vi "HOST Serial thruster update.vi"(8 "error in (no error)":errorcluster, 11 "Data out":T1={"VI References"=[], "Addresses"=[], "Pilot"=FALSE, "DO Data"=[], "Access Restricted?"=FALSE, "Pilot Control References"=[], "CoPilot Control References"=[], "cRIO Config"=[], "datalog Q"=refnum, "PS_P"={"AI"=[], "DI"=[], "DO"=[], "Serial"=[], "CPU"={"Total Load"=[], "Interrupt Load"=[], "Total Physical"=0.0, "Free Physical"=0.0, "Primary Disk Capacity"=0.0, "Primary Disk Free"=0.0}, "Stop"=FALSE, "DO Channel"=[]}, "PS_S"={"AI"=[], "DI"=[], "DO"=[], "Serial"=[], "CPU"={"Total Load"=[], "Interrupt Load"=[], "Total Physical"=0.0, "Free Physical"=0.0, "Primary Disk Capacity"=0.0, "Primary Disk Free"=0.0}, "Stop"=FALSE, "DO Channel"=[]}, "IDE_P"={"AI"=[], "DI"=[], "DO"=[], "Serial"=[], "CPU"={"Total Load"=[], "Interrupt Load"=[], "Total Physical"=0.0, "Free Physical"=0.0, "Primary Disk Capacity"=0.0, "Primary Disk Free"=0.0}, "Stop"=FALSE, "DO Channel"=[]}, "IDE_S"={"AI"=[], "DI"=[], "DO"=[], "Serial"=[], "CPU"={"Total Load"=[], "Interrupt Load"=[], "Total Physical"=0.0, "Free Physical"=0.0, "Primary Disk Capacity"=0.0, "Primary Disk Free"=0.0}, "Stop"=FALSE, "DO Channel"=[]}, "PDE_P"={"AI"=[], "DI"=[], "DO"=[], "Serial"=[], "CPU"={"Total Load"=[], "Interrupt Load"=[], "Total Physical"=0.0, "Free Physical"=0.0, "Primary Disk Capacity"=0.0, "Primary Disk Free"=0.0}, "Stop"=FALSE, "DO Channel"=[]}, "PDE_S"={"AI"=[], "DI"=[], "DO"=[], "Serial"=[], "CPU"={"Total Load"=[], "Interrupt Load"=[], "Total Physical"=0.0, "Free Physical"=0.0, "Primary Disk Capacity"=0.0, "Primary Disk Free"=0.0}, "Stop"=FALSE, "DO Channel"=[]}, "GUI References"={"Control Names"=[], "Control References"=[]}, "GUI Data"=[], "TCP - Serial"=[], "TCP-Serial Q"=refnum, "TCP Serial Ref"=[], "Data Sets"=[], "Last Data"=[], "Alarm Data"=[], "DI Data"=[], "Ack Data"=[], "Buzzer Data"=[], "Pilot DO"=[], "Co-Pilot DO"=[], "System Down?"=FALSE, "Log Data"=[], "Update Array"=[], "MCC Data Log"=[], "MCC Data Not"=refnum, "Thruster control"=[refnum, refnum, refnum, refnum, refnum, refnum, refnum, refnum, refnum], "waga notifier out"=refnum, "Wago  log"=[], "Thruster Cont"=[0.0, 0.0, 0.0, 0.0, 0.0, 0.0, 0.0, 0.0, 0.0], "Cam Cont"=[FALSE, FALSE, FALSE, FALSE, FALSE, TRUE], "PDE_P TH Cont"={"COM 10"=0.0, "COM 11"=0.0, "COM 12"=0.0, "COM 13"=0.0}, "PDE_S TH Cont"={"COM 10"=0.0, "COM 11"=0.0, "COM 12"=0.0, "COM 13"=0.0}} {"cRIO Config"."AI"."Interface Data"."Timing"."sample mode" items=["Finite Samples"=10178, "Continuous Samples"=10123, "Hardware Timed Single Point"=12522]; "cRIO Config"."Async"."Interface Data"."Data"."Minor Frame Count" min=5 max=8 step=1}) -> (0 "error out":errorcluster, 3 "Data out 2":T1={"VI References"=[], "Addresses"=[], "Pilot"=FALSE, "DO Data"=[], "Access Restricted?"=FALSE, "Pilot Control References"=[], "CoPilot Control References"=[], "cRIO Config"=[], "datalog Q"=refnum, "PS_P"={"AI"=[], "DI"=[], "DO"=[], "Serial"=[], "CPU"={"Total Load"=[], "Interrupt Load"=[], "Total Physical"=0.0, "Free Physical"=0.0, "Primary Disk Capacity"=0.0, "Primary Disk Free"=0.0}, "Stop"=FALSE, "DO Channel"=[]}, "PS_S"={"AI"=[], "DI"=[], "DO"=[], "Serial"=[], "CPU"={"Total Load"=[], "Interrupt Load"=[], "Total Physical"=0.0, "Free Physical"=0.0, "Primary Disk Capacity"=0.0, "Primary Disk Free"=0.0}, "Stop"=FALSE, "DO Channel"=[]}, "IDE_P"={"AI"=[], "DI"=[], "DO"=[], "Serial"=[], "CPU"={"Total Load"=[], "Interrupt Load"=[], "Total Physical"=0.0, "Free Physical"=0.0, "Primary Disk Capacity"=0.0, "Primary Disk Free"=0.0}, "Stop"=FALSE, "DO Channel"=[]}, "IDE_S"={"AI"=[], "DI"=[], "DO"=[], "Serial"=[], "CPU"={"Total Load"=[], "Interrupt Load"=[], "Total Physical"=0.0, "Free Physical"=0.0, "Primary Disk Capacity"=0.0, "Primary Disk Free"=0.0}, "Stop"=FALSE, "DO Channel"=[]}, "PDE_P"={"AI"=[], "DI"=[], "DO"=[], "Serial"=[], "CPU"={"Total Load"=[], "Interrupt Load"=[], "Total Physical"=0.0, "Free Physical"=0.0, "Primary Disk Capacity"=0.0, "Primary Disk Free"=0.0}, "Stop"=FALSE, "DO Channel"=[]}, "PDE_S"={"AI"=[], "DI"=[], "DO"=[], "Serial"=[], "CPU"={"Total Load"=[], "Interrupt Load"=[], "Total Physical"=0.0, "Free Physical"=0.0, "Primary Disk Capacity"=0.0, "Primary Disk Free"=0.0}, "Stop"=FALSE, "DO Channel"=[]}, "GUI References"={"Control Names"=[], "Control References"=[]}, "GUI Data"=[], "TCP - Serial"=[], "TCP-Serial Q"=refnum, "TCP Serial Ref"=[], "Data Sets"=[], "Last Data"=[], "Alarm Data"=[], "DI Data"=[], "Ack Data"=[], "Buzzer Data"=[], "Pilot DO"=[], "Co-Pilot DO"=[], "System Down?"=FALSE, "Log Data"=[], "Update Array"=[], "MCC Data Log"=[], "MCC Data Not"=refnum, "Thruster control"=[refnum, refnum, refnum, refnum, refnum, refnum, refnum, refnum, refnum], "waga notifier out"=refnum, "Wago  log"=[], "Thruster Cont"=[0.0, 0.0, 0.0, 0.0, 0.0, 0.0, 0.0, 0.0, 0.0], "Cam Cont"=[FALSE, FALSE, FALSE, FALSE, FALSE, TRUE], "PDE_P TH Cont"={"COM 10"=0.0, "COM 11"=0.0, "COM 12"=0.0, "COM 13"=0.0}, "PDE_S TH Cont"={"COM 10"=0.0, "COM 11"=0.0, "COM 12"=0.0, "COM 13"=0.0}} {"cRIO Config"."AI"."Interface Data"."Timing"."sample mode" items=["Finite Samples"=10178, "Continuous Samples"=10123, "Hardware Timed Single Point"=12522]; "cRIO Config"."Async"."Interface Data"."Data"."Minor Frame Count" min=5 max=8 step=1})   [LabVIEW 2021]
doc: "Thruster control data trnsmission to teh slave will be updated with this Vi. The data will be read from the serial and updated with corresponding to Slave and System Down Status."
uses:
  Controls/Host - GUI Data Cluster.ctl
  Analog Output/Controls/AO JSON Data Cluster.ctl
  Analog Output/Controls/AO Interface Data Cluster.ctl
  Analog Output/Controls/AO Channel Configuration Cluster.ctl
  Analog Output/Controls/AO Timing Cluster.ctl
  Digital Output/Controls/DIO Configuration cluster.ctl
  Digital Output/Controls/DIO Interface Data.ctl
  Digital Output/SubVIs/Digital Dynamic Cluster.ctl
  Async JSON Cluster.ctl
  Async Interface Data Cluster.ctl
  Async Serial/Controls/Async Serial Configuration Cluster.ctl
  Async Serial/Controls/Async Frame Info Cluster.ctl
  Async Serial/Controls/Async Message Info Cluster.ctl
  Controls/Host Data Cluster.ctl
  Main Engine/Controls/Main Engine CPU Info.ctl
panel:
  out "PDE_S.Serial 2":string[][](array[string])
  out "Array":i32[](array[numeric])
  out "PDE_S.Serial":string[][](array[string])=[["com21", "4000.000000", "TRUE", "", "", "", "", "", "", "", "", ""], ["com12", "96.000000", "156.989250", "0.125000", "37.678600", "28.353846", "-138.261345", "19.484347", "0.000000", "0.000000", "0.000000", "0.000000"], ["com13", "96.000000", "157.038750", "0.750000", "37.678025", "28.353846", "21.753627", "19.979010", "0.000000", "0.000000", "0.000000", "0.000000"], ["com10", "96.000000", "157.088250", "0.250000", "37.677450", "31.169231", "22.048668", "20.077840", "0.000000", "0.000000", "0.000000", "0.000000"], ["com11", "96.000000", "157.830750", "0.250000", "37.679175", "30.856410", "20.670168", "20.176638", "0.000000", "0.000000", "0.000000", "0.000000"]]
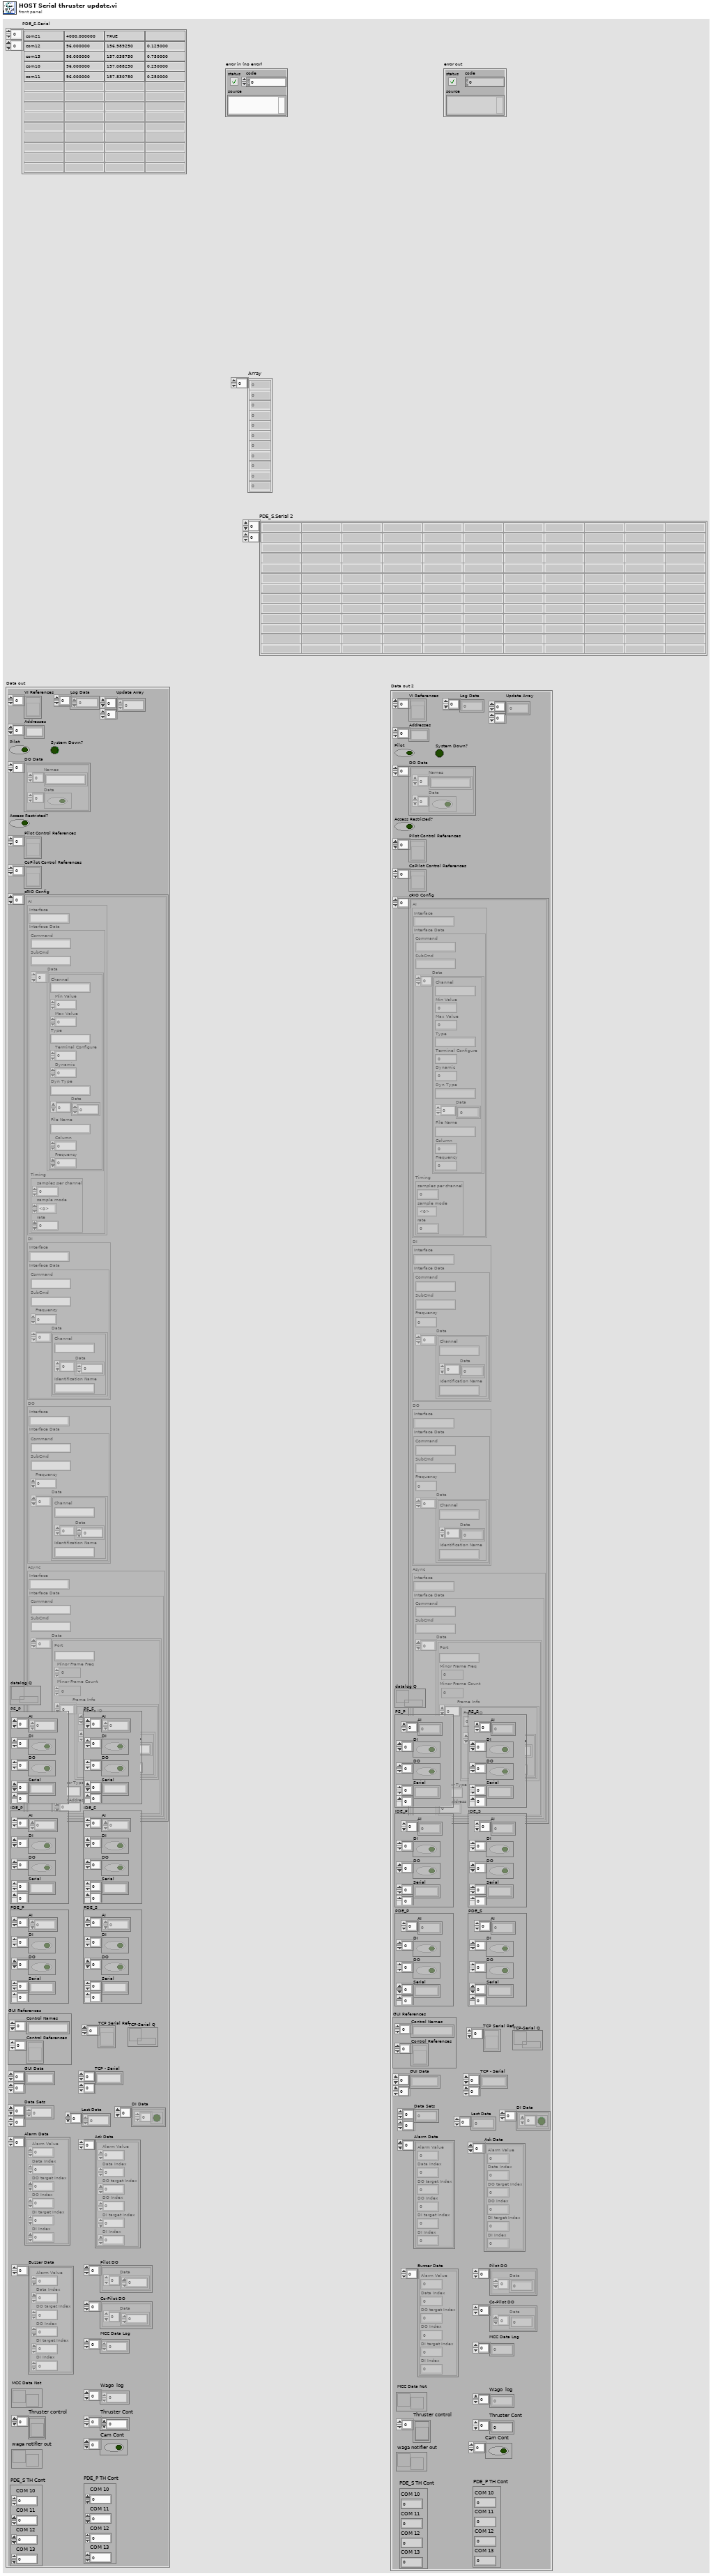
[diagram p1: front panel]
types:
  T1 = typedef "Host - GUI Data Cluster.ctl" = cluster{"VI References":refnum<vi>[], "Addresses":string[], "Pilot":bool, "DO Data":cluster{"Names":string[], "Data":bool[]}[], "Access Restricted?":bool, "Pilot Control References":refnum<vi>[], "CoPilot Control References":refnum<vi>[], "cRIO Config":cluster{"AI":T2, "DI":T6, "DO":T6, "Async":T9}[], "datalog Q":refnum<queue>, "PS_P":T14, "PS_S":T14, "IDE_P":T14, "IDE_S":T14, "PDE_P":T14, "PDE_S":T14, "GUI References":cluster{"Control Names":string[], "Control References":refnum<vi>[]}, "GUI Data":string[][], "TCP - Serial":string[][], "TCP-Serial Q":refnum<queue>, "TCP Serial Ref":refnum<vi>[], "Data Sets":dbl[][], "Last Data":dbl[], "Alarm Data":cluster{"Alarm Value":dbl, "Data Index":i32, "DO target Index":i32, "DO Index":i32, "DI target Index":i32, "DI Index":i32}[], "DI Data":cluster{bool[]}[], "Ack Data":cluster{"Alarm Value":dbl, "Data Index":i32, "DO target Index":i32, "DO Index":i32, "DI target Index":i32, "DI Index":i32}[], "Buzzer Data":cluster{"Alarm Value":dbl, "Data Index":i32, "DO target Index":i32, "DO Index":i32, "DI target Index":i32, "DI Index":i32}[], "Pilot DO":cluster{"Data":i32[]}[], "Co-Pilot DO":cluster{"Data":i32[]}[], "System Down?":bool, "Log Data":dbl[], "Update Array":i32[][], "MCC Data Log":dbl[], "MCC Data Not":refnum<notifier>, "Thruster control":refnum<vi>[], "waga notifier out":refnum<notifier>, "Wago  log":sgl[], "Thruster Cont":dbl[], "Cam Cont":bool[], "PDE_P TH Cont":cluster{"COM 10":dbl, "COM 11":dbl, "COM 12":dbl, "COM 13":dbl}, "PDE_S TH Cont":cluster{"COM 10":dbl, "COM 11":dbl, "COM 12":dbl, "COM 13":dbl}}
  T2 = typedef "AO JSON Data Cluster.ctl" = cluster{"Interface":string, "Interface Data":T3}
  T3 = typedef "AO Interface Data Cluster.ctl" = cluster{"Command":string, "SubCmd":string, "Data":T4[], "Timing":T5}
  T4 = typedef "AO Channel Configuration Cluster.ctl" = cluster{"Channel":string, "Min Value":dbl, "Max Value":dbl, "Type":string, "Terminal Configure":u16, "Dynamic":u8, "Dyn Type":string, "Data":dbl[], "File Name":string, "Column":i32, "Frequency":dbl}
  T5 = typedef "AO Timing Cluster.ctl" = cluster{"samples per channel":i32, "sample mode":i32, "rate":dbl}
  T6 = typedef "DIO Configuration cluster.ctl" = cluster{"Interface":string, "Interface Data":T7}
  T7 = typedef "DIO Interface Data.ctl" = cluster{"Command":string, "SubCmd":string, "Frequency":u16, "Data":T8[]}
  T8 = typedef "Digital Dynamic Cluster.ctl" = cluster{"Channel":string, "Data":u8[], "Identification Name":string}
  T9 = typedef "Async JSON Cluster.ctl" = cluster{"Interface":string, "Interface Data":T10}
  T10 = typedef "Async Interface Data Cluster.ctl" = cluster{"Command":string, "SubCmd":string, "Data":T11[]}
  T11 = typedef "Async Serial Configuration Cluster.ctl" = cluster{"Port":string, "Minor Frame Freq":u16, "Minor Frame Count":u16, "Frame Info":T12[], "Sensor Type":u16, "OIM Address":u16}
  T12 = typedef "Async Frame Info Cluster.ctl" = cluster{"Frame ID":u16, "Message Info":T13[]}
  T13 = typedef "Async Message Info Cluster.ctl" = cluster{"Message":u8[], "Message Name":string}
  T14 = typedef "Host Data Cluster.ctl" = cluster{"AI":dbl[], "DI":bool[], "DO":bool[], "Serial":string[][], "CPU":T15, "Stop":bool, "DO Channel":string[]}
  T15 = typedef "Main Engine CPU Info.ctl" = cluster{"Total Load":u32[], "Interrupt Load":u32[], "Total Physical":dbl, "Free Physical":dbl, "Primary Disk Capacity":dbl, "Primary Disk Free":dbl}
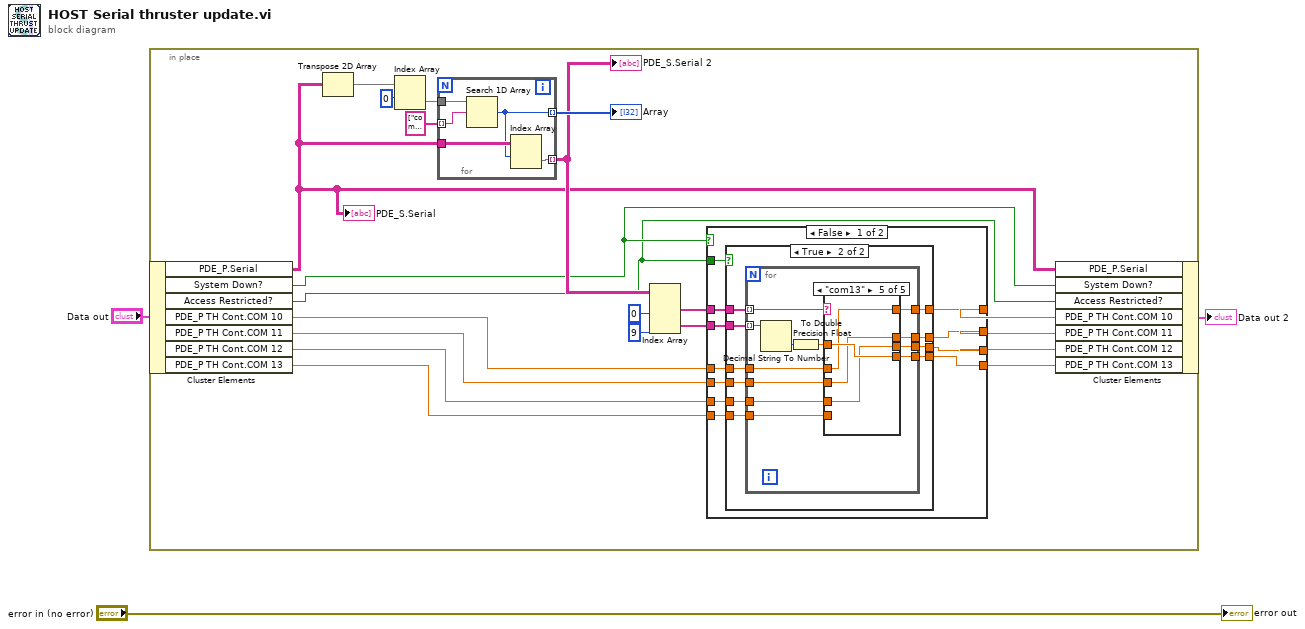
[diagram p0: block diagram]
diagram:
  n1 = in-place {
    n2 = in-place-cluster #1("Data out") -> ("PDE_P.Serial"=w7:string[][], "System Down?"=w6:bool, "Access Restricted?"=w5:bool, "PDE_P TH Cont.COM 10"=w20:dbl, "PDE_P TH Cont.COM 11"=w19:dbl, "PDE_P TH Cont.COM 12"=w18:dbl, "PDE_P TH Cont.COM 13"=w17:dbl)
    "PDE_S.Serial" <- w7
    n3 = Transpose 2D Array(2D array=w7) -> (transposed array=w11:string[][])
    n4 = Index Array(array=w11, index (row)=0) -> (element=w9:string[])  [unwired: 1 in]
    n5 = for {
      tunnel: string[] ["com10", "com11", "com12", "com13"] -> [w25] mode=indexing
      tunnel: [w28] -> w12 mode=indexing
      tunnel: w7 -> [w29]
      tunnel: [w27] -> w8 mode=indexing
      tunnel: w9 -> [w26]
      n6 = Search 1D Array(1D array=w26, element=w25) -> (index of element=w28:i32)  [unwired: 1 in]
      n7 = Index Array(array=w29, index (row)=w28) -> (element=w27:string[])  [unwired: 1 in]
    }
    "Array" <- w12
    "PDE_S.Serial 2" <- w8
    n8 = Index Array(array=w8, index (col) #1=0 ("disabled index (col)"), index (col) #2=9 ("index (col)")) -> (element #1=w22:string[], element #2=w21:string[])  [unwired: 2 in]
    n9 = case shown="False" w6 {
      tunnel: w5 -> [w40 _]
      tunnel: w22 -> [w39 _]
      tunnel: w21 -> [w38 _]
      tunnel: w20 -> [w37 w90]
      tunnel: w19 -> [w36 w89]
      tunnel: w18 -> [w35 w88]
      tunnel: w17 -> [w34 w87]
      tunnel: [w33 w90] -> w4
      tunnel: [w32 w89] -> w16
      tunnel: [w31 w88] -> w15
      tunnel: [w30 w87] -> w14
      frame False {
        n10 = case shown="True" w40 {
          tunnel: w39 -> [_ w54]
          tunnel: w38 -> [_ w53]
          tunnel: w37 -> [w44 w52]
          tunnel: w36 -> [w43 w51]
          tunnel: w35 -> [w42 w50]
          tunnel: w34 -> [w41 w49]
          tunnel: [w44 w48] -> w33
          tunnel: [w43 w47] -> w32
          tunnel: [w42 w46] -> w31
          tunnel: [w41 w45] -> w30
          frame False {
          }
          frame True {
            n11 = for {
              tunnel: w54 -> [w66] mode=indexing
              tunnel: w53 -> [w65] mode=indexing
              tunnel: [w62] -> w46
              tunnel: [w61] -> w48
              tunnel: [w60] -> w47
              tunnel: [w59] -> w45
              tunnel: w52 -> [w58]
              tunnel: w51 -> [w57]
              tunnel: w50 -> [w56]
              tunnel: w49 -> [w55]
              n12 = Decimal String To Number(string=w65) -> (number=w64:i32)  [unwired: 2 in, 1 out]
              n13 = To Double Precision Float(number=w64) -> (double precision float=w63:dbl)
              n14 = case shown="\"com13\"" w66 {
                tunnel: w63 -> [_ w74 w78 w80 w86]
                tunnel: [w68 w72 w76 w80 w83] -> w62
                tunnel: [w70 w74 w77 w82 w85] -> w61
                tunnel: [w69 w73 w78 w81 w84] -> w60
                tunnel: [w67 w71 w75 w79 w86] -> w59
                tunnel: w58 -> [w70 _ w77 w82 w85]
                tunnel: w57 -> [w69 w73 _ w81 w84]
                tunnel: w56 -> [w68 w72 w76 _ w83]
                tunnel: w55 -> [w67 w71 w75 w79 _]
                frame Default {
                }
                frame "com10" {
                }
                frame "com11" {
                }
                frame "com12" {
                }
                frame "com13" {
                }
              }
            }
          }
        }
      }
      frame True {
      }
    }
    n15 = in-place-cluster #1("PDE_P.Serial"=w7, "System Down?"=w6, "Access Restricted?"=w5, "PDE_P TH Cont.COM 10"=w4, "PDE_P TH Cont.COM 11"=w16, "PDE_P TH Cont.COM 12"=w15, "PDE_P TH Cont.COM 13"=w14) -> (→"Data out 2":T1)
  }
  "error out" <- "error in (no error)"
